vi "Add To Router.vi"(2 "niInstr AXI4-Lite address space collection v1 FPGA in":refnum<class "niInstr AXI4-Lite Address Space Collection v1 FPGA.lvclass">, 5 "Router in":refnum<class "Router.lvclass">) -> (6 "Router out":refnum<class "Router.lvclass">)   [LabVIEW 2015, in "niInstr AXI4-Lite Address Space Collection v1 FPGA.lvclass"]
doc: "Adds the Address Space Collection to the specified Router.\n\n<B>Input Parameters</B>\n\n<B>niInstr AXI4-Lite address space collection v1 FPGA in</B> is a reference to the Address Space Collection passed in from the previous VI.\n\n<B>Router in</B> is the Instruction Framework Router to which to add the passed in Address Space Collection.\n\n<B>Output Parameters</B>\n\n<B>Router out</B> passes the Instruction Framework Router to the next VI."
uses:
  <instrlib>/_niInstr/CLIP Adapters/v1/FPGA/AXI4-Lite/Address Space Collection/niInstr AXI4-Lite Address Space Collection v1 FPGA.lvclass
  <instrlib>/_niInstr/Instruction Framework/v1/FPGA/Interfaces/Router/Router.lvclass
  <instrlib>/_niInstr/CLIP Adapters/v1/FPGA/AXI4-Lite/Address Space Collection/niInstr AXI4-Lite Address Space Collection v1 FPGA.lvclass/niInstr AXI4-Lite Address Space Collection v1 FPGA.ctl
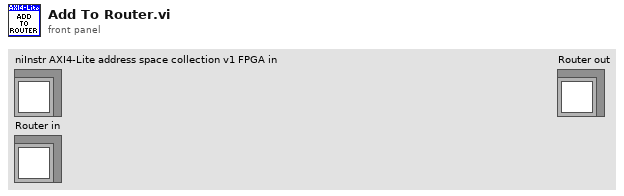
[diagram p1: front panel]
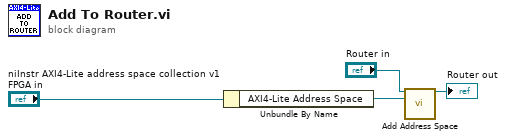
[diagram p0: block diagram]
diagram:
  n1 = Unbundle By Name("niInstr AXI4-Lite address space collection v1 FPGA in") -> ("AXI4-Lite Address Space"=w1:refnum<class "niInstr AXI4-Lite Address Space v1 FPGA.lvclass">)
  n2 = call-dynamic "Add Address Space.vi"("router in"="Router in", "address space"=w1) -> ("router out"=→"Router out":refnum<class "Router.lvclass">)  [unwired: 13 in]
